vi "Server.vi"() -> ()   [LabVIEW 2018]
uses:
  <vilib>/DAQmx/read.llb/DAQmx Read (Counter DBL 1Chan 1Samp).vi
  <vilib>/DAQmx/read.llb/DAQmx Read (Analog 1D Wfm NChan NSamp).vi
  <vilib>/DAQmx/create/channels.llb/DAQmx Create Channel (CI-Position-Angular Encoder).vi
  <vilib>/DAQmx/create/channels.llb/DAQmx Create Channel (AI-Voltage-Basic).vi
  <vilib>/DAQmx/configure/timing.llb/DAQmx Timing (Sample Clock).vi
  <vilib>/DAQmx/miscellaneous.llb/DAQmx Fill In Error Info.vi
  <vilib>/measure/macond.llb/IIR Filter for 1 Chan.vi
  <vilib>/Utility/file.llb/Write Delimited Spreadsheet (string).vi
  <vilib>/measure/NI_MAPro.lvlib
panel:
  in  "decoding type":i32(ring)=10090 items=["X1"=10090, "X2"=10091, "X4"=10092, "Two Pulse Counting"=10313]
  in  "pulses per revolution":u32=120
  in  "stop":bool
  in  "maximum value":dbl=5.0
  in  "minimum value":dbl=-5.0
  in  "Sensor Sensitivity (mV/g)":i32=289
  in  "port":u16=6340
  in  "Physical Channel":tag
  in  "IIR filter specifications 2":T1={"Topology"=enum."Butterworth", "Type"=enum."Lowpass", "Order"=3, "Lower Fc"=100.0, "Upper Fc"=200.0, "PB Ripple"=1.0, "SB Attenuation"=60.0} {"PB Ripple" format="%0.2f"; "SB Attenuation" format="%0.2f"; "Lower Fc" format="%0.2p"; "Upper Fc" format="%0.2p"}
  in  "Client Closed":string="The client VI closed the connection."
  out "Number of Samples":dbl=2000.0
  out "Sample Rate":dbl=1000.0
  out "Counter":tag="myDAQ1/ctr0"
  out "Analog Physical Channel 1":tag="myDAQ1/ai0"
  out "Analog Physical Channel 2":tag="myDAQ1/ai1"
  out "file path (dialog if empty)":path
  out "Waveform Graph":waveform(dbl)(graph)
  out "ai1 g Waveform Graph 2":waveform(dbl)(graph)
  out "ai0 g Waveform Graph 2":waveform(dbl)(graph)
  out "ai0 X-axis Waveform Graph":waveform(dbl)[](graph)
  out "IIR filter specifications":T1={"Topology"=enum."Butterworth", "Type"=enum."Lowpass", "Order"=3, "Lower Fc"=100.0, "Upper Fc"=200.0, "PB Ripple"=1.0, "SB Attenuation"=60.0} {"PB Ripple" format="%0.2f"; "SB Attenuation" format="%0.2f"; "Lower Fc" format="%0.2p"; "Upper Fc" format="%0.2p"}
  out "ai1 Y-axis Waveform Graph":waveform(dbl)[](graph)
  # "MEE 5318 Project 4 Server.vi\nGroup: 7\nMembers: Sagar Jagtap (903935334)\n                   Arunkumar Ramachandran (903928488)"
  # "Comm Settings"
  # "Channel Settings"
  # "Timing Settings"
  # "Analog Settings"
  # "Encoder Settings"
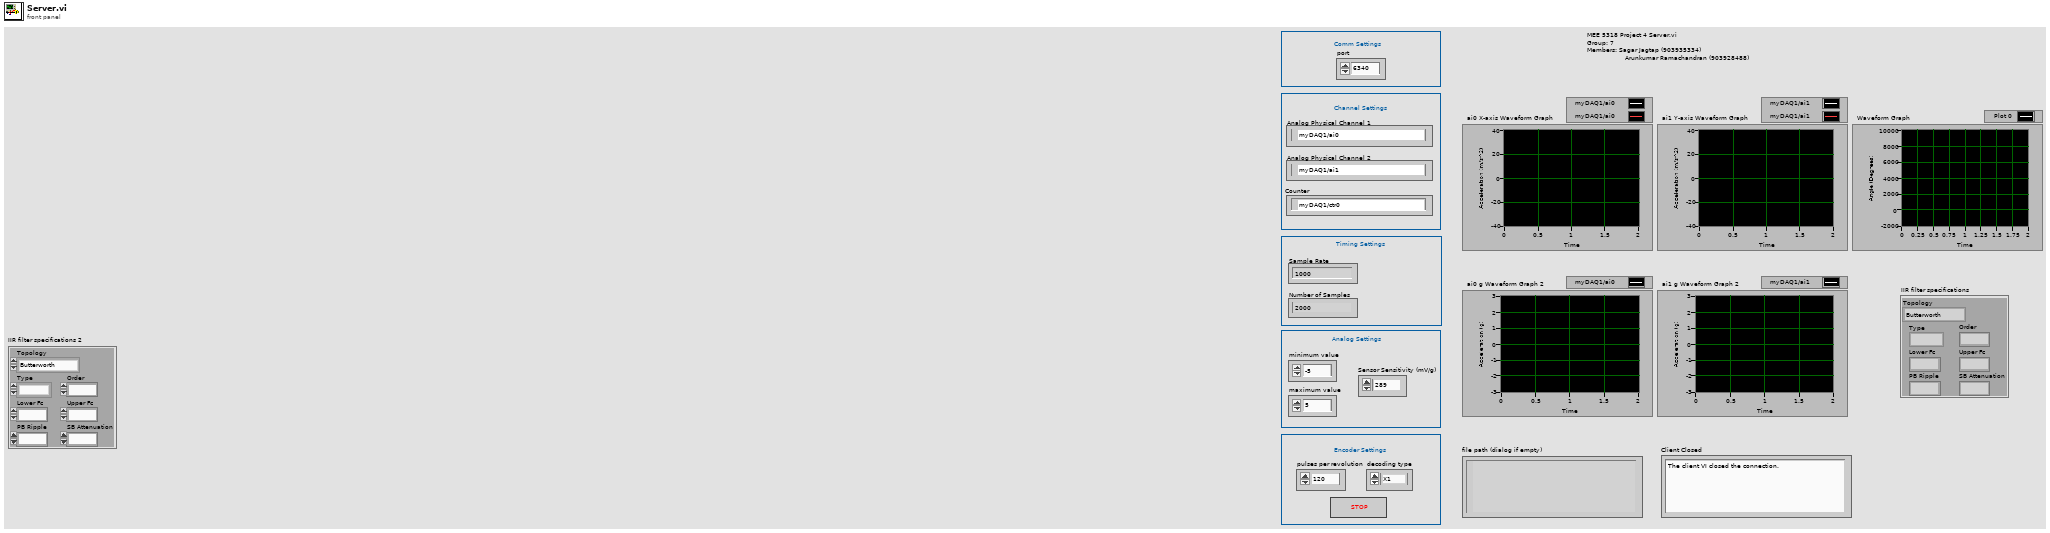
[diagram p1: front panel]
types:
  T1 = cluster{"Topology":enum16{"Off", "Butterworth", "Chebyshev", "Inverse Chebyshev", "Elliptic", "Bessel"}, "Type":enum16{"Lowpass", "Highpass", "Bandpass", "Bandstop"}, "Order":i32, "Lower Fc":dbl, "Upper Fc":dbl, "PB Ripple":dbl, "SB Attenuation":dbl}
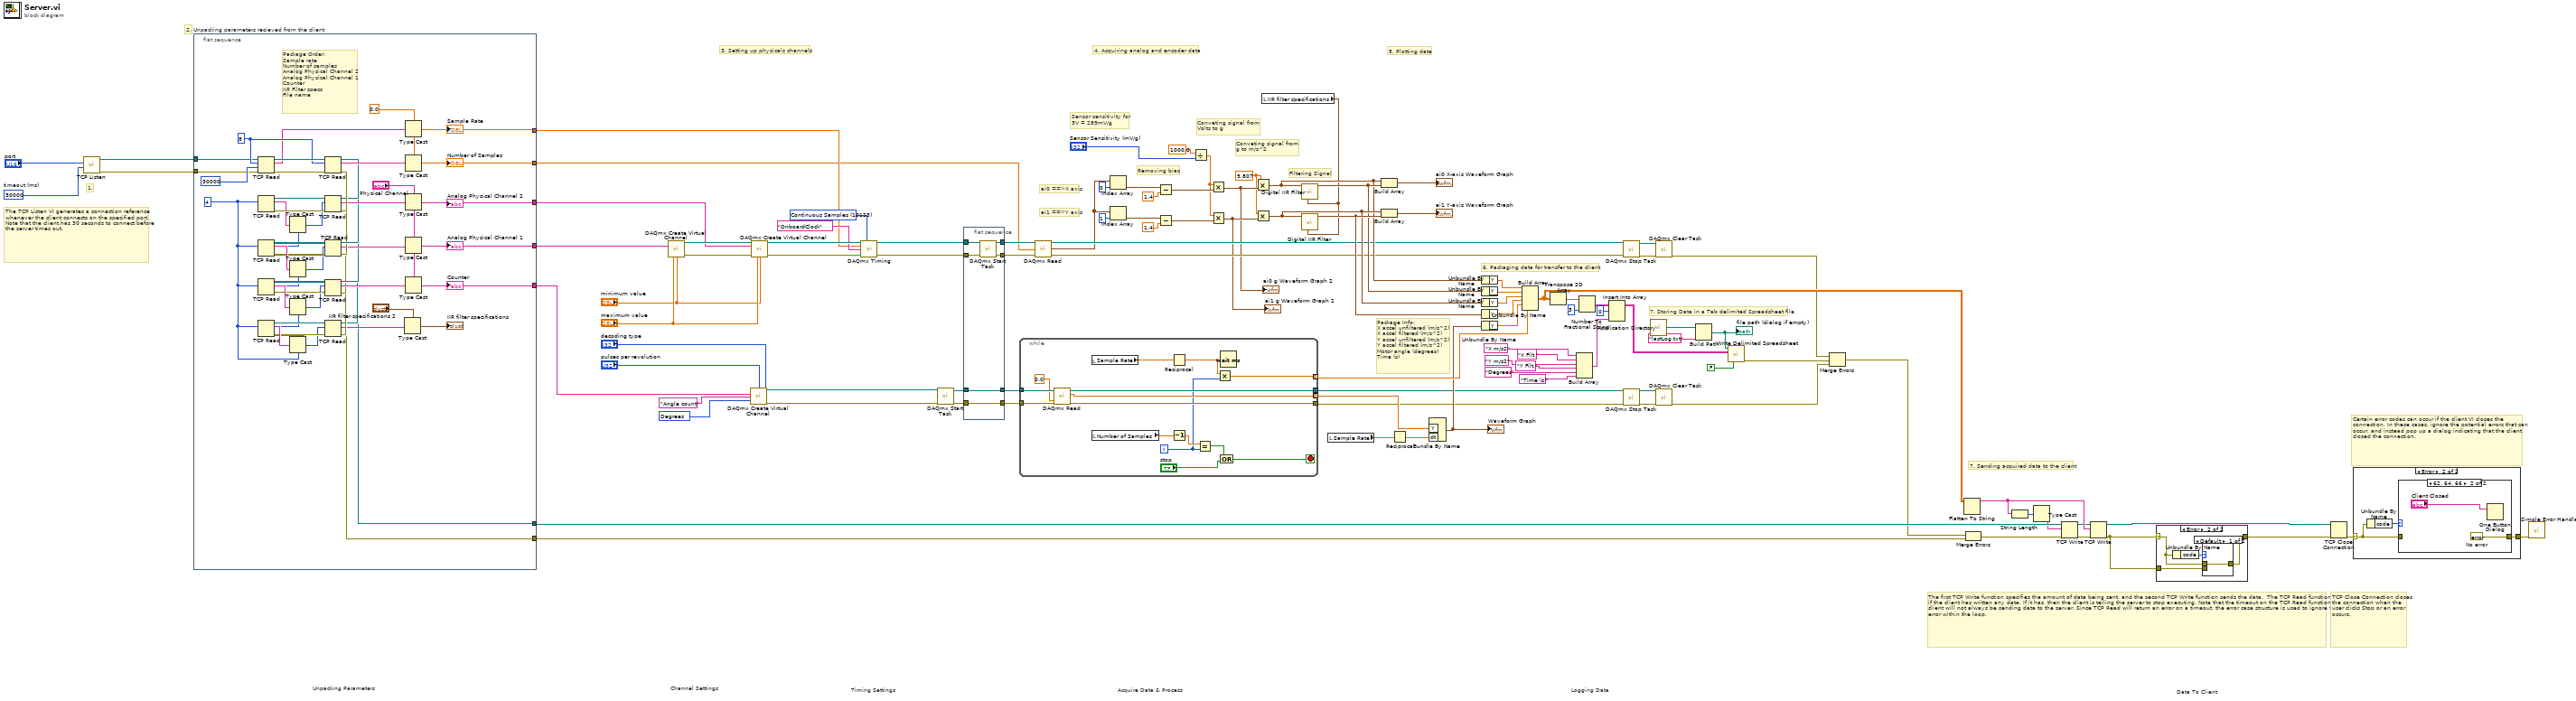
[diagram p0: block diagram]
diagram:
  w23 = 9.807 ("x")
  w14 = 10146 items=["Degrees"=10146, "Radians"=10273, "Ticks"=10304, "From Custom Scale"=10065] ("units")
  w17 = 10123 items=["Finite Samples"=10178, "Continuous Samples"=10123, "Hardware Timed Single Point"=12522] ("sample mode")
  w104 = 30000  # timeout (ms)
  # "7. Sending acquired data to the client"
  # "7. Storing Data in a Tab delimited Spreadsheet file"
  # "5. Plotting data"
  # "Package Info:\nX accel unfiltered (m/s^2)\nX accel filtered (m/s^2)\nY accel unfiltered (m/s^2)\nY accel filtered (m/s^2)\nMotor angle (degrees)\nTime (s)"
  # "Data To Client"
  # "4. Acquiring analog and encoder data"
  # "3. Setting up physicals channels"
  # "2."
  # "1."
  # "Unpacking Parameters"
  # "TCP Close Connection closes the connection when the user clicks Stop or an error occurs."
  # "Certain error codes can occur if the client VI closes the connection. In these cases, ignore the potential errors that can occur, and instead pop up a dialog indicating that the client closed the connection."
  # "The first TCP Write function specifies the amount of data being sent, and the second TCP Write function sends the data.  The TCP Read function checks to see if the client has written any data. If it has, then the client is telling the server to stop executing. Note that the timeout on the TCP Read function is '0', as the client will not always be sending data to the server. Since TCP Read will return an error on a timeout, the error case structure is used to ignore the timeout error within the loop."
  # "Logging Data"
  # "Acquire Data & Process"
  # "Timing Settings"
  # "Channel Settings"
  # "6. Packaging data for transfer to the client"
  # "ai1 ==>Y axis"
  # "ai0 ==>X axis"
  # "Filtering Signal"
  # "Conveting signal from\ng to m/s^2"
  # "Sensor sensitivity for\n3V = 289mV/g"
  # "Conveting signal from\nVolts to g"
  # "Removing bias"
  # "The TCP Listen VI generates a connection reference whenever the client connects on the specified port. Note that the client has 30 seconds to connect before the server times out."
  n1 = call <vilib>:"TCP Listen.vi"("timeout ms (wait forever: -1)"=w104, "port"="port") -> ("error out"=w102:errorcluster, "connection ID"=w103:refnum<k5>)  [unwired: 5 in, 3 out]
  n2 = flat-sequence "Unpacking parameters recieved from the client" {
    tunnel: [w106] -> w7
    tunnel: [w107] -> w105
    tunnel: w103 -> [w117]
    tunnel: w102 -> [w116]
    tunnel: [w113] -> w13
    tunnel: [w112] -> w12
    tunnel: [w111] -> w11
    tunnel: [w110] -> w10
    tunnel: [w109] -> w9
    frame #0 {
      w114 = 4 ("bytes to read")
      w150 = 0.0
      w149 = 8 ("bytes to read")
      # "Package Order:\nSample rate\nNumber of samples\nAnalog Physical Channel 2\nAnalog Physical Channel 1\nCounter\nIIR Filter specs\nFile name"
      n3 = TCP Read(connection ID=w117, bytes to read=w149, error in (no error)=w116, 9:30000 ("timeout ms (25000)")) -> (connection ID out=w152:refnum<k5>, data out=w148:string, error out=w151:errorcluster)  [unwired: 1 in]
      n4 = TCP Read(connection ID=w152, bytes to read=w149, error in (no error)=w151) -> (connection ID out=w145:refnum<k5>, data out=w147:string, error out=w146:errorcluster)  [unwired: 2 in]
      n5 = TCP Read(connection ID=w145, bytes to read=w114, error in (no error)=w146) -> (connection ID out=w143:refnum<k5>, data out=w144:string, error out=w142:errorcluster)  [unwired: 2 in]
      n6 = Type Cast(type=w114, x=w144) -> (*(type *) &x=w141:i32)
      n7 = TCP Read(connection ID=w143, bytes to read=w141, error in (no error)=w142) -> (connection ID out=w135:refnum<k5>, data out=w140:string, error out=w134:errorcluster)  [unwired: 2 in]
      n8 = TCP Read(connection ID=w135, bytes to read=w114, error in (no error)=w134) -> (connection ID out=w138:refnum<k5>, data out=w139:string, error out=w137:errorcluster)  [unwired: 2 in]
      n9 = Type Cast(type=w114, x=w139) -> (*(type *) &x=w136:i32)
      n10 = TCP Read(connection ID=w138, bytes to read=w136, error in (no error)=w137) -> (connection ID out=w127:refnum<k5>, data out=w133:string, error out=w126:errorcluster)  [unwired: 2 in]
      n11 = TCP Read(connection ID=w127, bytes to read=w114, error in (no error)=w126) -> (connection ID out=w131:refnum<k5>, data out=w132:string, error out=w130:errorcluster)  [unwired: 2 in]
      n12 = Type Cast(type=w114, x=w132) -> (*(type *) &x=w129:i32)
      n13 = TCP Read(connection ID=w131, bytes to read=w129, error in (no error)=w130) -> (connection ID out=w120:refnum<k5>, data out=w128:string, error out=w121:errorcluster)  [unwired: 2 in]
      n14 = TCP Read(connection ID=w120, bytes to read=w114, error in (no error)=w121) -> (connection ID out=w124:refnum<k5>, data out=w125:string, error out=w123:errorcluster)  [unwired: 2 in]
      n15 = Type Cast(type=w114, x=w125) -> (*(type *) &x=w122:i32)
      n16 = TCP Read(connection ID=w124, bytes to read=w122, error in (no error)=w123) -> (connection ID out=w107:refnum<k5>, data out=w119:string, error out=w106:errorcluster)  [unwired: 2 in]
      n17 = Type Cast(type="IIR filter specifications 2", x=w119) -> (*(type *) &x=→"IIR filter specifications":T1)
      n18 = Type Cast(type=w150, x=w148) -> (*(type *) &x=w111:dbl)
      "Sample Rate" <- w111
      n19 = Type Cast(type=w150, x=w147) -> (*(type *) &x=w110:dbl)
      "Number of Samples" <- w110
      n20 = Type Cast(type="Physical Channel", x=w140) -> (*(type *) &x=w113:tag)
      "Analog Physical Channel 2" <- w113
      n21 = Type Cast(type="Physical Channel", x=w133) -> (*(type *) &x=w112:tag)
      "Analog Physical Channel 1" <- w112
      n22 = Type Cast(type="Physical Channel", x=w128) -> (*(type *) &x=w109:tag)
      "Counter" <- w109
    }
  }
  n23 = call-poly <vilib>:"DAQmx Create Virtual Channel.vi"("maximum value"="maximum value", "minimum value"="minimum value", "physical channels"=w12) -> ("task out"=w44:refnum<k21>, "error out"=w45:errorcluster)  [unwired: 11 in]
  n24 = call-poly <vilib>:"DAQmx Create Virtual Channel.vi"("counter"=w9, "decoding type"="decoding type", "name to assign"="Angle count", "units"=w14, "pulses per revolution"="pulses per revolution") -> ("task out"=w39:refnum<k21>, "error out"=w40:errorcluster)  [unwired: 9 in]
  n25 = call-poly <vilib>:"DAQmx Create Virtual Channel.vi"("task in"=w44, "maximum value"="maximum value", "minimum value"="minimum value", "physical channels"=w13, "error in"=w45) -> ("task out"=w46:refnum<k21>, "error out"=w47:errorcluster)  [unwired: 9 in]
  n26 = call-poly <vilib>:"DAQmx Timing.vi"("task/channels in"=w46, "sample mode"=w17, "rate"=w11, "source"=tag "OnboardClock", "error in"=w47) -> ("task out"=w37:refnum<k21>, "error out"=w38:errorcluster)  [unwired: 9 in]
  n27 = call <vilib>:"DAQmx Start Task.vi"("task/channels in"=w39, "error in"=w40) -> ("task out"=w86:refnum<k21>, "error out"=w88:errorcluster)  [unwired: 12 in]
  n28 = flat-sequence {
    tunnel: w37 -> [w159]
    tunnel: w38 -> [w158]
    tunnel: [w157] -> w56
    tunnel: [w156] -> w57
    tunnel: w86 -> [w155]
    tunnel: [w155] -> w87
    tunnel: w88 -> [w154]
    tunnel: [w154] -> w89
    frame #0 {
      n29 = call <vilib>:"DAQmx Start Task.vi"("task/channels in"=w159, "error in"=w158) -> ("task out"=w157:refnum<k21>, "error out"=w156:errorcluster)  [unwired: 12 in]
    }
  }
  n30 = while {
    tunnel: w87 -> [w174]
    tunnel: w89 -> [w173]
    tunnel: [w172] -> w41
    tunnel: [w171] -> w42
    tunnel: [w167] -> w72 mode=indexing
    tunnel: [w162] -> w79 mode=indexing
    i -> [w163]
    stop <- w169 stop-if-true
    n31 = call-poly <vilib>:"DAQmx Read.vi"("task/channels in"=w174, "timeout"=0.0, "error in"=w173) -> ("task out"=w172:refnum<k21>, "data"=w167:dbl, "error out"=w171:errorcluster)  [unwired: 10 in]
    n32 = local read "Sample Rate"() -> (w161:dbl)
    n33 = local read "Number of Samples"() -> (w164:dbl)
    n34 = Reciprocal(x=w161) -> (1/x=w160:dbl)
    n35 = Decrement(x=w164) -> (x-1=w165:dbl)
    n36 = Equal?(x=w165, y=w163) -> (x = y?=w168:bool)
    n37 = Multiply(x=w160, y=w163) -> (x*y=w162:dbl)
    n38 = Wait (ms)(milliseconds to wait=w160) -> ()  [unwired: 1 out]
    n39 = Compound Arithmetic op=OR(w168, "stop") -> (w169:bool)
  }
  n40 = call-poly <vilib>:"DAQmx Read.vi"("task/channels in"=w56, "number of samples per channel"=w10, "error in"=w57) -> ("task out"=w59:refnum<k21>, "data"=w54:waveform(dbl)[], "error out"=w60:errorcluster)  [unwired: 10 in]
  n41 = Index Array(array=w54, index=0) -> (element=w53:waveform(dbl))
  n42 = Index Array(array=w54, index=1) -> (element=w51:waveform(dbl))
  n43 = Subtract(x=w53, y=1.4) -> (x-y=w55:waveform(dbl))
  n44 = Subtract(x=w51, y=1.4) -> (x-y=w52:waveform(dbl))
  n45 = Divide(x=1000.0, y="Sensor Sensitivity (mV/g)") -> (x/y=w50:dbl)
  n46 = Multiply(x=w50, y=w55) -> (x*y=w48:waveform(dbl))
  "ai0 g Waveform Graph 2" <- w48
  n47 = Multiply(x=w50, y=w52) -> (x*y=w58:waveform(dbl))
  "ai1 g Waveform Graph 2" <- w58
  n48 = Multiply(x=w23, y=w48) -> (x*y=w63:waveform(dbl))
  n49 = Multiply(x=w23, y=w58) -> (x*y=w65:waveform(dbl))
  n50 = local read "IIR filter specifications"() -> (w8:T1)
  n51 = call-poly <vilib>:"Digital IIR Filter.vi"("IIR filter specifications"=w8, "signal in"=w63) -> ("signal out"=w64:waveform(dbl))  [unwired: 7 in, 2 out]
  n52 = call-poly <vilib>:"Digital IIR Filter.vi"("IIR filter specifications"=w8, "signal in"=w65) -> ("signal out"=w66:waveform(dbl))  [unwired: 7 in, 2 out]
  n53 = local read "Sample Rate"() -> (w62:dbl)
  n54 = Build Array(w63, w64) -> (→"ai0 X-axis Waveform Graph":waveform(dbl)[])
  n55 = Build Array(w65, w66) -> (→"ai1 Y-axis Waveform Graph":waveform(dbl)[])
  n56 = Reciprocal(x=w62) -> (1/x=w61:dbl)
  n57 = Bundle By Name("Y"=w72, "dt"=w61) -> (w67:waveform(dbl))  [unwired: 1 in]
  "Waveform Graph" <- w67
  n58 = Unbundle By Name(w63) -> ("Y"=w73:dbl[])
  n59 = Unbundle By Name(w64) -> ("Y"=w68:dbl[])
  n60 = Unbundle By Name(w65) -> ("Y"=w69:dbl[])
  n61 = Unbundle By Name(w66) -> ("Y"=w70:dbl[])
  n62 = Unbundle By Name(w67) -> ("Y"=w71:dbl[])
  n63 = Build Array(w73, w68, w69, w70, w71, w79) -> (w100:dbl[][])
  n64 = Transpose 2D Array(2D array=w100) -> (transposed array=w98:dbl[][])
  n65 = Build Array("X m/s2", "X Filt.", "Y m/s2", "Y Filt.", "Degrees", "Time (s)") -> (w81:string[])
  n66 = Number To Fractional String(number=w98, precision (6)=i16 3) -> (F-format string=w80:string[][])  [unwired: 2 in]
  n67 = Insert Into Array(array=w80, index (row)=0, new element=w81) -> (w82:string[][])  [unwired: 1 in]
  n68 = call <vilib>:"DAQmx Stop Task.vi"("task/channels in"=w59, "error in"=w60) -> ("task out"=w33:refnum<k21>, "error out"=w34:errorcluster)  [unwired: 12 in]
  n69 = call <vilib>:"DAQmx Stop Task.vi"("task/channels in"=w41, "error in"=w42) -> ("task out"=w36:refnum<k21>, "error out"=w35:errorcluster)  [unwired: 12 in]
  n70 = call <vilib>:"Application Directory.vi"() -> ("Application Directory"=w4:path)
  n71 = call <vilib>:"DAQmx Clear Task.vi"("task in"=w33, "error in"=w34) -> ("error out"=w43:errorcluster)  [unwired: 13 in]
  n72 = call <vilib>:"DAQmx Clear Task.vi"("task in"=w36, "error in"=w35) -> ("error out"=w77:errorcluster)  [unwired: 13 in]
  n73 = Build Path(base path=w4, name or relative path="lastLog.txt") -> (appended path=w2:path)
  "file path (dialog if empty)" <- w2
  n74 = call-poly <vilib>:"Write Delimited Spreadsheet.vi"("file path (dialog if empty)"=w2, "2D data"=w82, "transpose? (no:F)"=FALSE) -> ("error out"=w78:errorcluster)  [unwired: 11 in, 1 out]
  n75 = Merge Errors(w43, w78, w77) -> (w5:errorcluster)
  n76 = Flatten To String(anything=w100) -> (data string=w99:string)  [unwired: 3 in, 2 out]
  n77 = Merge Errors(w5, w7) -> (w6:errorcluster)
  n78 = String Length(string=w99) -> (length=w95:i32)
  n79 = Type Cast(x=w95) -> (*(type *) &x=w101:string)  [unwired: 1 out]
  n80 = TCP Write(connection ID=w105, data in=w101, error in (no error)=w6) -> (connection ID out=w93:refnum<k5>, error out=w94:errorcluster)  [unwired: 2 out]
  n81 = TCP Write(connection ID=w93, data in=w99, error in (no error)=w94) -> (connection ID out=w96:refnum<k5>, error out=w97:errorcluster)  [unwired: 2 out]
  n82 = case shown="Error" w97 {
    selector: w97 -> [w175 w178]
    tunnel: [w175 w176] -> w90
    tunnel: w97 -> [_ w177]
    frame No Error {
    }
    frame Error {
      n83 = Unbundle By Name(w178) -> ("code"=w179:i32)
      n84 = case shown="Default" w179 {
        tunnel: w178 -> [w180 _]
        tunnel: w177 -> [_ w181]
        tunnel: [w180 w181] -> w176
        frame Default {
        }
        frame 56 {
        }
      }
    }
  }
  n85 = TCP Close Connection(connection ID=w96, error in (no error)=w90) -> (error out=w91:errorcluster)  [unwired: 2 out]
  n86 = case shown="Error" w91 {
    selector: w91 -> [w182 w184]
    tunnel: [w182 w183] -> w92
    frame No Error {
    }
    frame Error {
      n87 = Unbundle By Name(w184) -> ("code"=w185:i32)
      n88 = case shown="62, 64, 66" w185 {
        tunnel: w184 -> [w186 _]
        tunnel: [w186 w188] -> w183
        frame Default {
        }
        frame 62, 64, 66 {
          w188 = errorcluster {"status"=FALSE, "code"=0, "source"=""}  # No error
          n89 = One Button Dialog(message="Client Closed") -> ()  [unwired: 1 in, 1 out]
        }
      }
    }
  }
  n90 = call <vilib>:"Simple Error Handler.vi"("error in (no error)"=w92) -> ()  [unwired: 1 in, 8 out]
